vi "Teleop.vi"(10 "Match Info":T1={"Autonomous Elapsed Seconds"=0.0, "TeleOp Elapsed Seconds"=0.0, "Disabled Elapsed Seconds"=0.0, "Visited Autonomous"=FALSE, "Visited TeleOp"=FALSE, "Visited Disabled"=FALSE, "Autonomous Settings"={"Autonomous Style"=enum."Independent", "VI Refnum"=refnum}}, 11 "Call Context":T2) -> ()   [LabVIEW 2013]
doc: "This VI is called for each TeleOp packet received from the DS where the robot is not disabled. It is often used to read from the joysticks and update I/O or to update setpoints for timed control loops. It should complete and return within 20 milliseconds or it may miss DS packets."
uses:
  <vilib>/Rock Robotics/WPI/DriverStation/WPI_DriverStationDerivedRobotMode.ctl
  <vilib>/Rock Robotics/WPI/DriverStation/WPI_DriverStationMatch Info.ctl
  <vilib>/Rock Robotics/WPI/DriverStation/DriverStationLCD/WPI_DriverStationLCDLCDLine.ctl
  Robot Global Data.vi
  <vilib>/Rock Robotics/WPI/RobotDrive/WPI_RobotDriveArcadeDrive_Standard(NoSaturation).vi
  <vilib>/Rock Robotics/WPI/Joystick/WPI_JoystickGetSetRefNum.vi
  <vilib>/Rock Robotics/WPI/Solenoid/Deprecated/WPI_SolenoidSetBool.vi
  <vilib>/Rock Robotics/WPI/RobotDrive/WPI_RobotDriveGetSetRefNum.vi
panel:
  out "Numeric 1":dbl(slide) scale=0.0..100.0
  out "Boolean 2":bool
  out "Boolean 1":bool
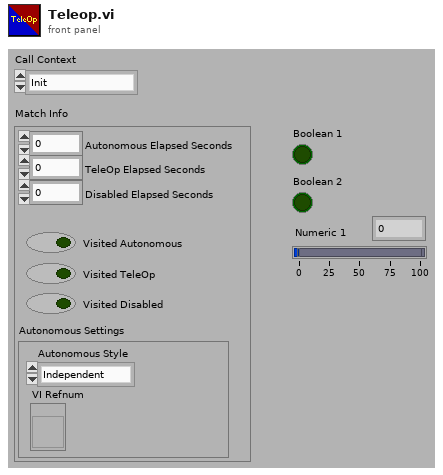
[diagram p1: front panel]
types:
  T1 = typedef "WPI_DriverStationMatch Info.ctl" = cluster{"Autonomous Elapsed Seconds":dbl, "TeleOp Elapsed Seconds":dbl, "Disabled Elapsed Seconds":dbl, "Visited Autonomous":bool, "Visited TeleOp":bool, "Visited Disabled":bool, "Autonomous Settings":cluster{"Autonomous Style":enum16{"Iterative", "Independent"}, "VI Refnum":refnum<vi>}}
  T2 = typedef "WPI_DriverStationDerivedRobotMode.ctl" = enum16{"Init", "Execute", "Stop"}
  T3 = typedef "WPI_DriverStationLCDLCDLine.ctl" = enum16{"Main - Line 1", "User - Line 2", "User - Line 3", "User - Line 4", "User - Line 5", "User - Line 6"}
  T4 = typedef "WPI_DigitalInputDevRef.ctl" = cluster{"DevStatus":errorcluster, "DIO Channel":T5, "Digital Module":T6}
  T5 = typedef "FPGA_DIOChannel.ctl" = enum8{"DIO 1", "DIO 2", "DIO 3", "DIO 4", "DIO 5", "DIO 6", "DIO 7", "DIO 8", "DIO 9", "DIO 10", "DIO 11", "DIO 12", "DIO 13", "DIO 14", "Invalid"}
  T6 = typedef "FPGA_TypedefDigitalModule.ctl" = enum16{"Digital Module 1", "Digital Module 2"}
  T7 = typedef "WPI_JoystickDevRef.ctl" = cluster{"Device":T8}
  T8 = typedef "WPI_JoystickDeviceEnum.ctl" = enum16{"USB 1", "USB 2", "USB 3", "USB 4", "Kinect 1", "Kinect 2"}
  T9 = typedef "WPI_JoystickButtonState.ctl" = cluster{"Button 1":bool, "Button 2":bool, "Button 3":bool, "Button 4":bool, "Button 5":bool, "Button 6":bool, "Button 7":bool, "Button 8":bool, "Button 9":bool, "Button 10":bool, "Button 11":bool, "Button 12":bool}
  T10 = cluster{"axis 1 (x)":dbl, "axis 2 (y)":dbl, "axis 3 (throttle)":dbl, "axis 4":dbl, "axis 5":dbl, "axis 6":dbl}
  T11 = typedef "WPI_MotorControlDeviceRef.ctl" = cluster{"DeviceStatus":errorcluster, "Type":enum16{"PWM", "CAN"}, "PWM":cluster{"Digital Module":T6, "PWM Channel":T12, "DeadBand":T13}, "CAN":cluster{"Device Number":u8, "Control Mode":T14, "Semaphore":T15, "Max Vout":dbl}, "Invert":bool, "TransformRef":T16, "InvTransformRef":T16}
  T12 = typedef "FPGA_DIOPWMChannel.ctl" = enum8{"PWM 1", "PWM 2", "PWM 3", "PWM 4", "PWM 5", "PWM 6", "PWM 7", "PWM 8", "PWM 9", "PWM 10", "Invalid"}
  T13 = typedef "WPI_PWMDeadband.ctl" = cluster{"Name":string, "maxPositivePwm":i32, "minPositivePwm":i32, "centerPwm":i32, "maxNegativePwm":i32, "minNegativePwm":i32, "angularRange":u16}
  T14 = typedef "WPI_CANJaguar_ControlMode.ctl" = enum8{"Percent VBus", "Current", "Speed", "Position", "Voltage"}
  T15 = typedef "Semaphore RefNum" = refnum<k1>
  T16 = typedef "WPI_PWMTransform_ConPane.ctl" = refnum<vi>
  T17 = typedef "WPI_SolenoidDevRef.ctl" = cluster{"DevStatus":errorcluster, "Solenoid Module":T18, "Forward Solenoid Channel":T19, "Reverse Solenoid Channel":T19}
  T18 = typedef "FPGA_TypedefSolenoidModule.ctl" = enum16{"Solenoid Module 1", "Solenoid Module 2"}
  T19 = typedef "WPI_SolenoidChannel.ctl" = enum8{"Solenoid 1", "Solenoid 2", "Solenoid 3", "Solenoid 4", "Solenoid 5", "Solenoid 6", "Solenoid 7", "Solenoid 8", "Invalid"}
  T20 = typedef "WPI_RobotDriveDevRef.ctl" = cluster{"DevStatus":errorcluster, "Motors[]":T11[], "Square Inputs":bool, "Max Output":dbl, "Isochronous":bool}
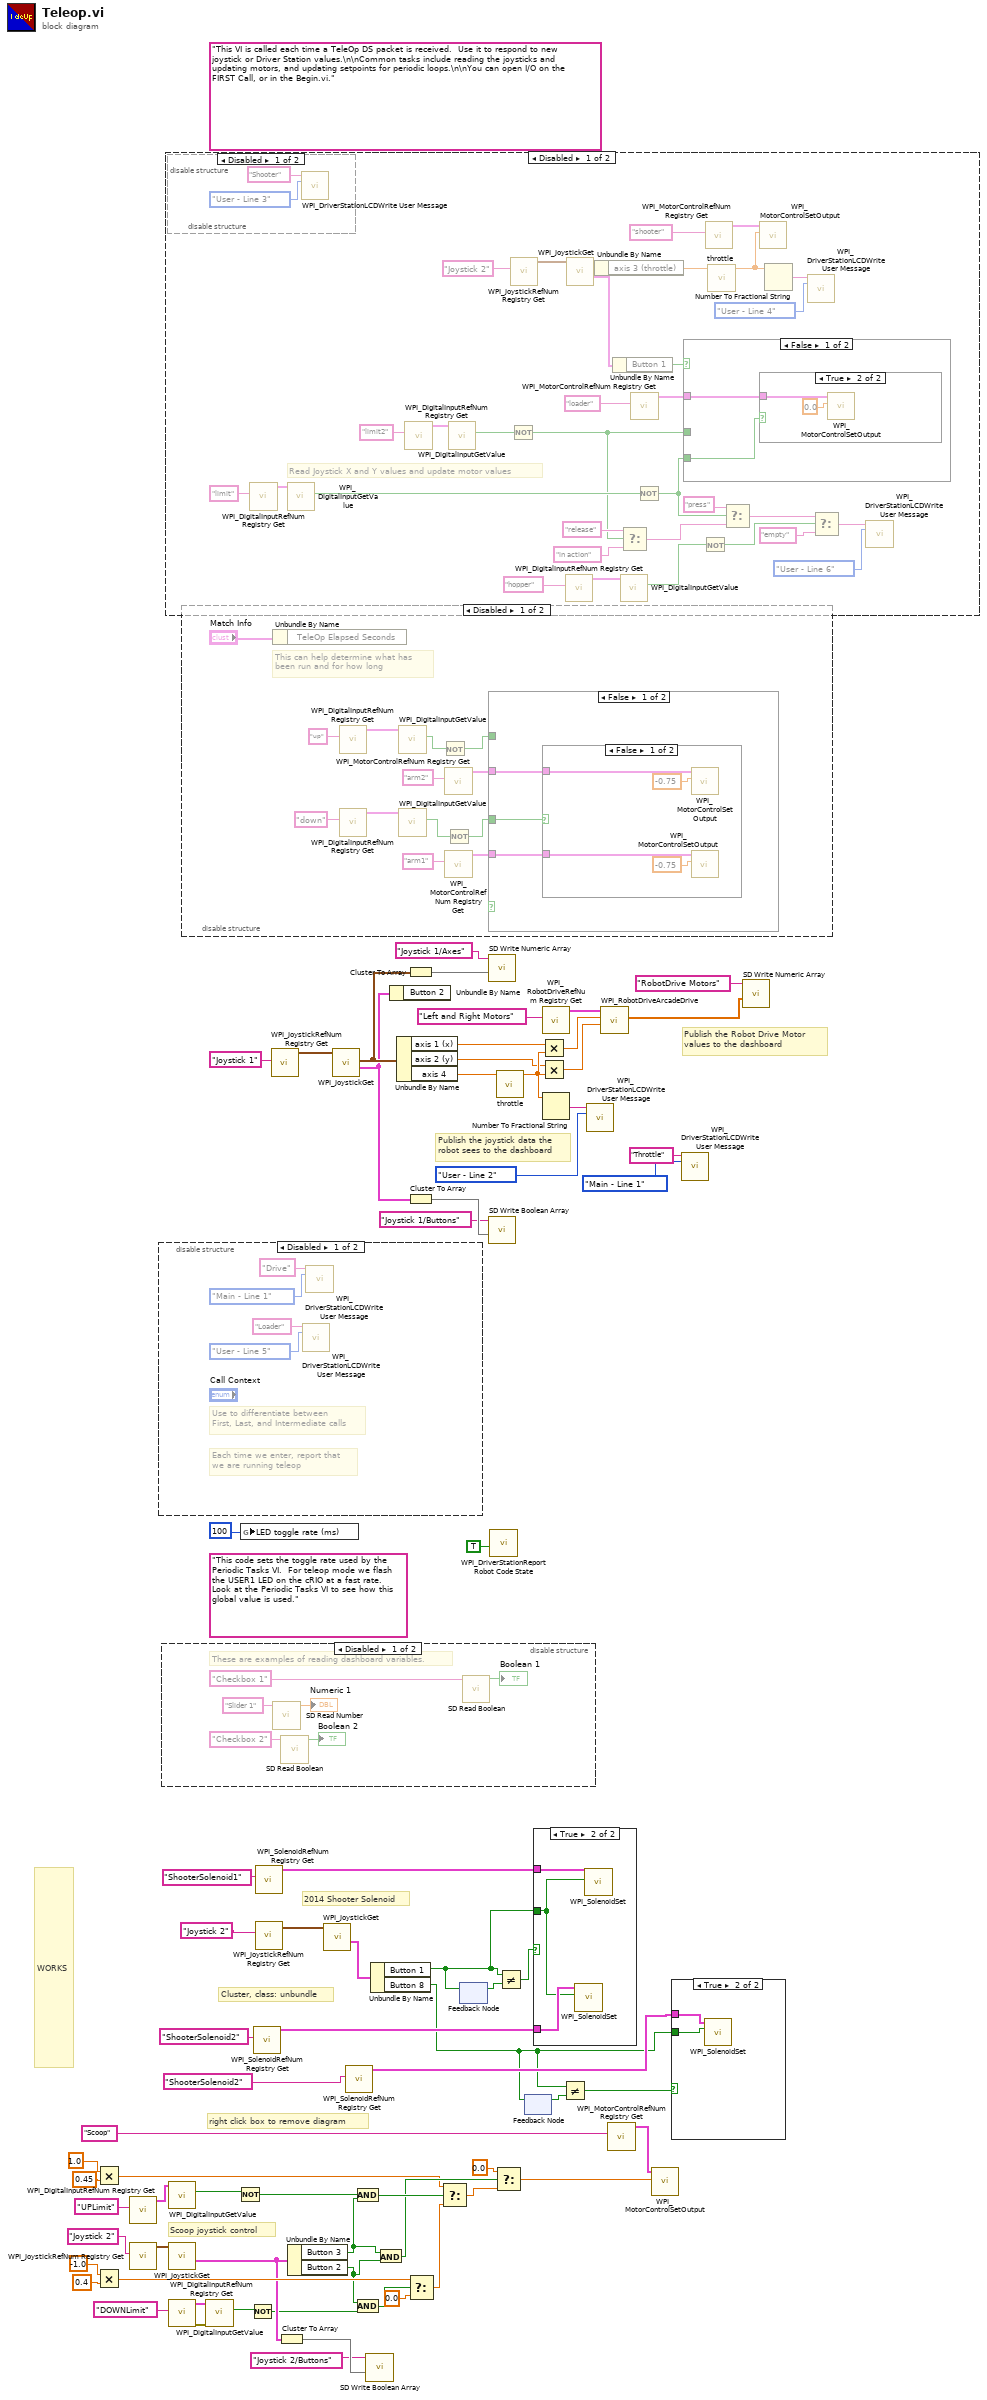
[diagram p0: block diagram]
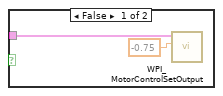
[diagram p3: hidden frame]
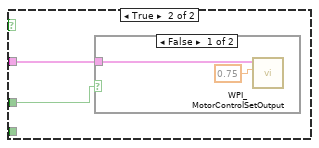
[diagram p4: hidden frame]
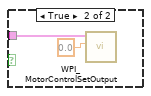
[diagram p5: hidden frame]
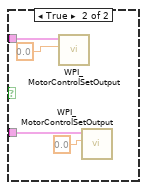
[diagram p11: hidden frame]
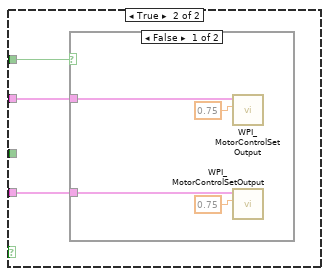
[diagram p12: hidden frame]
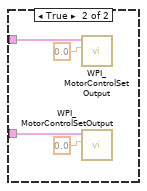
[diagram p13: hidden frame]
diagram:
  (unwired) "This code sets the toggle rate used by the Periodic Tasks VI.  For teleop mode we flash the USER1 LED on the cRIO at a fast rate.  Look at the Periodic Tasks VI to see how this global value is used."
  (unwired) "This VI is called each time a TeleOp DS packet is received.  Use it to respond to new joystick or Driver Station values.\n\nCommon tasks include reading the joysticks and updating motors, and updating setpoints for periodic loops.\n\nYou can open I/O on the FIRST Call, or in the Begin.vi."
  # "right click box to remove diagram"
  # "Scoop joystick control"
  # "WORKS"
  # "2014 Shooter Solenoid"
  # "Cluster, class: unbundle"
  # "Publish the Robot Drive Motor\nvalues to the dashboard"
  # "Publish the joystick data the\nrobot sees to the dashboard"
  n1 = Multiply(x=1.0, y=0.45) -> (x*y=w21:dbl)
  n2 = Multiply(x=-1.0, y=0.4) -> (x*y=w22:dbl)
  n3 = call <vilib>:"WPI_DigitalInputRefNum Registry Get.vi"("refnum name"="UPLimit") -> ("DigitalInputDevRef"=w36:T4)  [unwired: 9 in, 1 out]
  n4 = call <vilib>:"WPI_JoystickRefNum Registry Get.vi"("refnum name"="Joystick 2") -> ("JoystickDevRef"=w39:T7)  [unwired: 9 in, 1 out]
  n5 = disable-structure shown="Disabled" {
    frame Disabled {
      # "Each time we enter, report that\nwe are running teleop"
      # "Use to differentiate between\nFirst, Last, and Intermediate calls"
      n6 = call <vilib>:"WPI_DriverStationLCDWrite User Message.vi"("line text"="Loader", "line"=WPI_DriverStationLCDLCDLine."User - Line 5") -> ()  [unwired: 13 in, 1 out]
      n7 = call <vilib>:"WPI_DriverStationLCDWrite User Message.vi"("line text"="Drive", "line"=WPI_DriverStationLCDLCDLine."Main - Line 1") -> ()  [unwired: 13 in, 1 out]
    }
    frame Enabled {
    }
  }
  n8 = disable-structure shown="Disabled" {
    frame Disabled {
      # "These are examples of reading dashboard variables."
      n9 = call <vilib>:"SD Read Number.vi"("Name"="Slider 1" ("refnum name")) -> ("Numeric"=→"Numeric 1":dbl)  [unwired: 8 in, 2 out]
      n10 = call <vilib>:"SD Read Boolean.vi"("Name"="Checkbox 2" ("refnum name")) -> ("Boolean"=→"Boolean 2":bool)  [unwired: 8 in, 2 out]
      n11 = call <vilib>:"SD Read Boolean.vi"("Name"="Checkbox 1" ("refnum name")) -> ("Boolean"=→"Boolean 1":bool)  [unwired: 8 in, 2 out]
    }
    frame Enabled {
    }
  }
  n12 = disable-structure shown="Disabled" {
    frame Disabled {
      # "Read Joystick X and Y values and update motor values"
      n13 = disable-structure shown="Disabled" {
        frame Disabled {
          n14 = call <vilib>:"WPI_DriverStationLCDWrite User Message.vi"("line text"="Shooter", "line"=WPI_DriverStationLCDLCDLine."User - Line 3") -> ()  [unwired: 13 in, 1 out]
        }
        frame Enabled {
        }
      }
      n15 = call <vilib>:"WPI_DigitalInputRefNum Registry Get.vi"("refnum name"="limit") -> ("DigitalInputDevRef"=w111:T4)  [unwired: 9 in, 1 out]
      n16 = call <vilib>:"WPI_DigitalInputGetValue.vi"("DigitalInputDevRef"=w111) -> ("Value"=w105:bool)  [unwired: 8 in, 2 out]
      n17 = call <vilib>:"WPI_DigitalInputRefNum Registry Get.vi"("refnum name"="limit2") -> ("DigitalInputDevRef"=w107:T4)  [unwired: 9 in, 1 out]
      n18 = call <vilib>:"WPI_DigitalInputGetValue.vi"("DigitalInputDevRef"=w107) -> ("Value"=w106:bool)  [unwired: 8 in, 2 out]
      n19 = Not(x=w106) -> (.not. x?=w99:bool)
      n20 = call <vilib>:"WPI_JoystickRefNum Registry Get.vi"("refnum name"="Joystick 2") -> ("JoystickDevRef"=w97:T7)  [unwired: 1 in, 9 out]
      n21 = call <vilib>:"WPI_DigitalInputRefNum Registry Get.vi"("refnum name"="hopper") -> ("DigitalInputDevRef"=w87:T4)  [unwired: 9 in, 1 out]
      n22 = call <vilib>:"WPI_JoystickGet.vi"("JoystickDevRef"=w97) -> ("Buttons"=w94:T9, "Axes"=w95:T10)  [unwired: 1 in, 4 out]
      n23 = Unbundle By Name(w95) -> ("axis 3 (throttle)"=w93:dbl)
      n24 = Unbundle By Name(w94) -> ("Button 1"=w90:bool)
      n25 = call <vilib>:"WPI_DigitalInputGetValue.vi"("DigitalInputDevRef"=w87) -> ("Value"=w86:bool)  [unwired: 8 in, 2 out]
      n26 = Select(t="release", s=w99, f="in action") -> (s? t:f=w104:string)
      n27 = call <vilib>:"WPI_MotorControlRefNum Registry Get.vi"("refnum name"="loader") -> ("MotorControlDevRef"=w98:T11)  [unwired: 9 in, 1 out]
      n28 = Not(x=w105) -> (.not. x?=w100:bool)
      n29 = case shown="False" w90 {
        tunnel: w98 -> [w115 w121]
        tunnel: w99 -> [_ w122]
        tunnel: w100 -> [w116 _]
        frame False {
          n30 = case shown="True" w116 {
            tunnel: w115 -> [w117 w119]
            frame False {
              n31 = call <vilib>:"WPI_MotorControlSetOutput.vi"("Output"=-0.75, "MotorControlDevRef"=w117) -> ()  [unwired: 7 in, 3 out]
            }
            frame True {
              n32 = call <vilib>:"WPI_MotorControlSetOutput.vi"("Output"=0.0, "MotorControlDevRef"=w119) -> ()  [unwired: 7 in, 3 out]
            }
          }
        }
        frame True {
          n33 = case shown="False" w122 {
            tunnel: w121 -> [w124 w126]
            frame False {
              n34 = call <vilib>:"WPI_MotorControlSetOutput.vi"("Output"=0.75, "MotorControlDevRef"=w124) -> ()  [unwired: 7 in, 3 out]
            }
            frame True {
              n35 = call <vilib>:"WPI_MotorControlSetOutput.vi"("Output"=0.0, "MotorControlDevRef"=w126) -> ()  [unwired: 7 in, 3 out]
            }
          }
        }
      }
      n36 = Not(x=w86) -> (.not. x?=w83:bool)
      n37 = call <vilib>:"WPI_MotorControlRefNum Registry Get.vi"("refnum name"="shooter") -> ("MotorControlDevRef"=w114:T11)  [unwired: 9 in, 1 out]
      n38 = call "throttle.vi"("x"=w93) -> ("x/y"=w89:dbl)  [unwired: 10 in]
      n39 = Select(t="press", s=w100, f=w104) -> (s? t:f=w85:string)
      n40 = call <vilib>:"WPI_MotorControlSetOutput.vi"("Output"=w89, "MotorControlDevRef"=w114) -> ()  [unwired: 7 in, 3 out]
      n41 = Number To Fractional String(number=w89) -> (F-format string=w92:string)  [unwired: 3 in]
      n42 = call <vilib>:"WPI_DriverStationLCDWrite User Message.vi"("line text"=w92, "line"=WPI_DriverStationLCDLCDLine."User - Line 4") -> ()  [unwired: 13 in, 1 out]
      n43 = Select(t=w85, s=w83, f="empty") -> (s? t:f=w84:string)
      n44 = call <vilib>:"WPI_DriverStationLCDWrite User Message.vi"("line text"=w84, "line"=WPI_DriverStationLCDLCDLine."User - Line 6") -> ()  [unwired: 13 in, 1 out]
    }
    frame Enabled {
    }
  }
  n45 = call <vilib>:"WPI_DigitalInputGetValue.vi"("DigitalInputDevRef"=w36) -> ("Value"=w12:bool)  [unwired: 8 in, 2 out]
  n46 = call <vilib>:"WPI_JoystickGet.vi"("JoystickDevRef"=w39) -> ("Buttons"=w15:T9)  [unwired: 4 in, 2 out]
  n47 = call <vilib>:"WPI_DigitalInputRefNum Registry Get.vi"("refnum name"="DOWNLimit") -> ("error out"=w38:errorcluster, "DigitalInputDevRef"=w37:T4)  [unwired: 9 in]
  n48 = disable-structure shown="Disabled" {
    frame Disabled {
      # "This can help determine what has\nbeen run and for how long"
      n49 = Unbundle By Name("Match Info") -> ()  [unwired: 1 out]
      n50 = call <vilib>:"WPI_DigitalInputRefNum Registry Get.vi"("refnum name"="up") -> ("DigitalInputDevRef"=w140:T4)  [unwired: 9 in, 1 out]
      n51 = call <vilib>:"WPI_DigitalInputRefNum Registry Get.vi"("refnum name"="down") -> ("DigitalInputDevRef"=w139:T4)  [unwired: 9 in, 1 out]
      n52 = call <vilib>:"WPI_DigitalInputGetValue.vi"("DigitalInputDevRef"=w140) -> ("Value"=w132:bool)  [unwired: 8 in, 2 out]
      n53 = call <vilib>:"WPI_DigitalInputGetValue.vi"("DigitalInputDevRef"=w139) -> ("Value"=w130:bool)  [unwired: 8 in, 2 out]
      n54 = Not(x=w132) -> (.not. x?=w131:bool)
      n55 = call <vilib>:"WPI_MotorControlRefNum Registry Get.vi"("refnum name"="arm2") -> ("MotorControlDevRef"=w135:T11)  [unwired: 9 in, 1 out]
      n56 = call <vilib>:"WPI_MotorControlRefNum Registry Get.vi"("refnum name"="arm1") -> ("MotorControlDevRef"=w136:T11)  [unwired: 9 in, 1 out]
      n57 = Not(x=w130) -> (.not. x?=w129:bool)
      n58 = case shown="False" {
        selector: _ -> [_ _]
        tunnel: w131 -> [_ w155]
        tunnel: w129 -> [w144 _]
        tunnel: w136 -> [w143 w154]
        tunnel: w135 -> [w142 w153]
        frame False {
          n59 = case shown="False" w144 {
            tunnel: w143 -> [w146 w151]
            tunnel: w142 -> [w145 w150]
            frame False {
              n60 = call <vilib>:"WPI_MotorControlSetOutput.vi"("Output"=-0.75, "MotorControlDevRef"=w145) -> ()  [unwired: 7 in, 3 out]
              n61 = call <vilib>:"WPI_MotorControlSetOutput.vi"("Output"=-0.75, "MotorControlDevRef"=w146) -> ()  [unwired: 7 in, 3 out]
            }
            frame True {
              n62 = call <vilib>:"WPI_MotorControlSetOutput.vi"("Output"=0.0, "MotorControlDevRef"=w150) -> ()  [unwired: 7 in, 3 out]
              n63 = call <vilib>:"WPI_MotorControlSetOutput.vi"("Output"=0.0, "MotorControlDevRef"=w151) -> ()  [unwired: 7 in, 3 out]
            }
          }
        }
        frame True {
          n64 = case shown="False" w155 {
            tunnel: w154 -> [w157 w161]
            tunnel: w153 -> [w156 w160]
            frame False {
              n65 = call <vilib>:"WPI_MotorControlSetOutput.vi"("Output"=0.75, "MotorControlDevRef"=w156) -> ()  [unwired: 7 in, 3 out]
              n66 = call <vilib>:"WPI_MotorControlSetOutput.vi"("Output"=0.75, "MotorControlDevRef"=w157) -> ()  [unwired: 7 in, 3 out]
            }
            frame True {
              n67 = call <vilib>:"WPI_MotorControlSetOutput.vi"("Output"=0.0, "MotorControlDevRef"=w160) -> ()  [unwired: 7 in, 3 out]
              n68 = call <vilib>:"WPI_MotorControlSetOutput.vi"("Output"=0.0, "MotorControlDevRef"=w161) -> ()  [unwired: 7 in, 3 out]
            }
          }
        }
      }
    }
    frame Enabled {
    }
  }
  n69 = call <vilib>:"WPI_DigitalInputGetValue.vi"("error in (no error)"=w38, "DigitalInputDevRef"=w37) -> ("Value"=w14:bool)  [unwired: 7 in, 2 out]
  n70 = Not(x=w12) -> (.not. x?=w11:bool)
  n71 = global write "Robot Global Data.vi" "LED toggle rate (ms)"(u32 100 ("LED ms toggle rate")) -> ()
  n72 = Not(x=w14) -> (.not. x?=w13:bool)
  n73 = call <vilib>:"WPI_SolenoidRefNum Registry Get.vi"("refnum name"="ShooterSolenoid2") -> ("SolenoidDevRef"=w45:T17)  [unwired: 9 in, 1 out]
  n74 = call <vilib>:"WPI_SolenoidRefNum Registry Get.vi"("refnum name"="ShooterSolenoid1") -> ("SolenoidDevRef"=w49:T17)  [unwired: 9 in, 1 out]
  n75 = call <vilib>:"WPI_JoystickRefNum Registry Get.vi"("refnum name"="Joystick 2") -> ("JoystickDevRef"=w48:T7)  [unwired: 9 in, 1 out]
  n76 = call <vilib>:"WPI_JoystickRefNum Registry Get.vi"("refnum name"="Joystick 1") -> ("JoystickDevRef"=w69:T7)  [unwired: 1 in, 9 out]
  n77 = Cluster To Array(cluster=w15) -> (array=w17:bool[])
  n78 = Unbundle By Name(w15) -> ("Button 3"=w19:bool, "Button 2"=w18:bool)
  n79 = call <vilib>:"WPI_JoystickGet.vi"("JoystickDevRef"=w48) -> ("Buttons"=w7:T9)  [unwired: 4 in, 2 out]
  n80 = call <vilib>:"WPI_JoystickGet.vi"("JoystickDevRef"=w69) -> ("Buttons"=w51:T9, "Axes"=w65:T10)  [unwired: 1 in, 4 out]
  n81 = call <vilib>:"WPI_SolenoidRefNum Registry Get.vi"("refnum name"="ShooterSolenoid2") -> ("SolenoidDevRef"=w4:T17)  [unwired: 9 in, 1 out]
  n82 = And(x=w11, y=w19) -> (x .and. y?=w33:bool)
  n83 = And(x=w18, y=w13) -> (x .and. y?=w32:bool)
  n84 = call <vilib>:"SD Write Boolean Array.vi"("Boolean Array"=w17, "Name"="Joystick 2/Buttons") -> ()  [unwired: 8 in, 2 out]
  n85 = Unbundle By Name(w7) -> ("Button 1"=w42:bool, "Button 8"=w1:bool)
  n86 = And(x=w19, y=w18) -> (x .and. y?=w28:bool)
  n87 = Unbundle By Name(w51) -> ()  [unwired: 1 out]
  n88 = Unbundle By Name(w65) -> ("axis 1 (x)"=w58:dbl, "axis 2 (y)"=w52:dbl, "axis 4"=w60:dbl)
  n89 = Cluster To Array(cluster=w65) -> (array=w64:dbl[])
  n90 = Cluster To Array(cluster=w51) -> (array=w67:bool[])
  n91 = Select(t=w22, s=w32, f=0.0) -> (s? t:f=w26:dbl)
  n92 = Select(t=w21, s=w33, f=w26) -> (s? t:f=w30:dbl)
  n93 = feedback-in #1(w42) -> ()
  n94 = feedback #1() -> (w43:bool)  [unwired: 1 in]
  n95 = call <vilib>:"SD Write Numeric Array.vi"("Numeric Array"=w64, "Name"="Joystick 1/Axes") -> ()  [unwired: 8 in, 2 out]
  n96 = call <vilib>:"SD Write Boolean Array.vi"("Boolean Array"=w67, "Name"="Joystick 1/Buttons") -> ()  [unwired: 8 in, 2 out]
  n97 = call <vilib>:"WPI_DriverStationReport Robot Code State.vi"("TeleOp"=TRUE ("Autonomous")) -> ()  [unwired: 10 in, 1 out]
  n98 = Select(t=0.0, s=w28, f=w30) -> (s? t:f=w20:dbl)
  n99 = call "throttle.vi"("x"=w60) -> ("x/y"=w55:dbl)  [unwired: 10 in]
  n100 = Not Equal?(x=w42, y=w43) -> (x != y?=w44:bool)
  n101 = feedback #2() -> (w3:bool)  [unwired: 1 in]
  n102 = feedback-in #2(w1) -> ()
  n103 = case shown="True" w44 {
    tunnel: w49 -> [_ w166]
    tunnel: w45 -> [_ w165]
    tunnel: w42 -> [_ w164]
    frame False {
    }
    frame True {
      n104 = call-poly <vilib>:"WPI_SolenoidSet.vi"("Value"=w164, "SolenoidDevRef"=w165) -> ()  [unwired: 8 in, 2 out]
      n105 = call-poly <vilib>:"WPI_SolenoidSet.vi"("Value"=w164, "SolenoidDevRef"=w166) -> ()  [unwired: 8 in, 2 out]
    }
  }
  n106 = Multiply(x=w58, y=w55) -> (x*y=w57:dbl)
  n107 = Multiply(x=w52, y=w55) -> (x*y=w59:dbl)
  n108 = call <vilib>:"WPI_RobotDriveRefNum Registry Get.vi"("refnum name"="Left and Right Motors") -> ("RobotDriveDevRef"=w53:T20)  [unwired: 1 in, 9 out]
  n109 = Number To Fractional String(number=w55) -> (F-format string=w56:string)  [unwired: 3 in]
  n110 = Not Equal?(x=w1, y=w3) -> (x != y?=w2:bool)
  n111 = call <vilib>:"WPI_DriverStationLCDWrite User Message.vi"("line text"=w56, "line"=WPI_DriverStationLCDLCDLine."User - Line 2") -> ()  [unwired: 13 in, 1 out]
  n112 = call-poly <vilib>:"WPI_RobotDriveArcadeDrive.vi"("Y axis value"=w59, "X axis value"=w57, "RobotDriveDevRef"=w53) -> ("Motor Values"=w61:dbl[])  [unwired: 6 in, 2 out]
  n113 = call <vilib>:"WPI_MotorControlRefNum Registry Get.vi"("refnum name"="Scoop") -> ("MotorControlDevRef"=w40:T11)  [unwired: 9 in, 1 out]
  n114 = call <vilib>:"WPI_MotorControlSetOutput.vi"("Output"=w20, "MotorControlDevRef"=w40) -> ()  [unwired: 7 in, 3 out]
  n115 = case shown="True" w2 {
    tunnel: w4 -> [_ w168]
    tunnel: w1 -> [_ w167]
    frame False {
    }
    frame True {
      n116 = call-poly <vilib>:"WPI_SolenoidSet.vi"("Value"=w167, "SolenoidDevRef"=w168) -> ()  [unwired: 8 in, 2 out]
    }
  }
  n117 = call <vilib>:"WPI_DriverStationLCDWrite User Message.vi"("line text"="Throttle", "line"=WPI_DriverStationLCDLCDLine."Main - Line 1") -> ()  [unwired: 13 in, 1 out]
  n118 = call <vilib>:"SD Write Numeric Array.vi"("Numeric Array"=w61, "Name"="RobotDrive Motors") -> ()  [unwired: 8 in, 2 out]
